vi "Create TCP Connection Handler.vi"(5 "TCPConnectionHandler in":refnum<class "TCPConnectionHandler.lvclass">, 8 "error in (no error)":errorcluster, 10 "NbConnections":refnum<user-event>, 11 "ServerRequest":refnum<queue>) -> (0 "error out":errorcluster, 3 "TCPConnectionHandler out":refnum<class "TCPConnectionHandler.lvclass">)   [LabVIEW 2013, in "MQTT_TCP.lvlib" / "TCPConnectionHandler.lvclass"]
uses:
  TCPConnectionHandler.lvclass
  MQTT_Base/Base Class/Request -- cluster.ctl
  <vilib>/LabVIEW Open Source Project/MQTT Control Packets/Control Packets/ControlPacket/ControlPacket.lvclass
  MQTT_Base/Base Class/Response -- cluster.ctl
  TCPConnectionHandler.lvclass/TCPConnectionHandler.ctl
  MQTT_Base/Base Class/MQTT_Base.lvclass
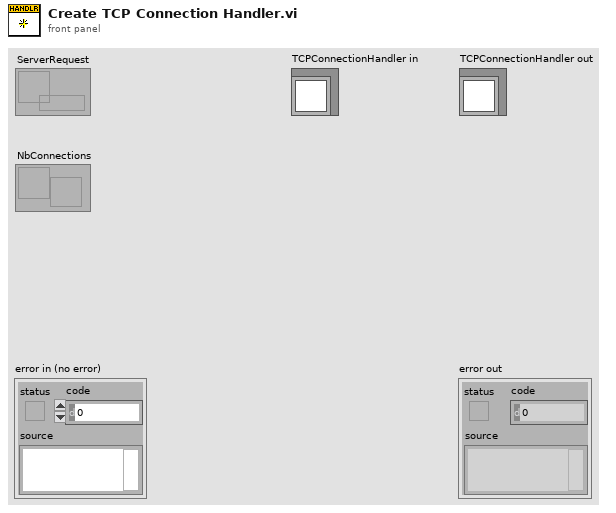
[diagram p1: front panel]
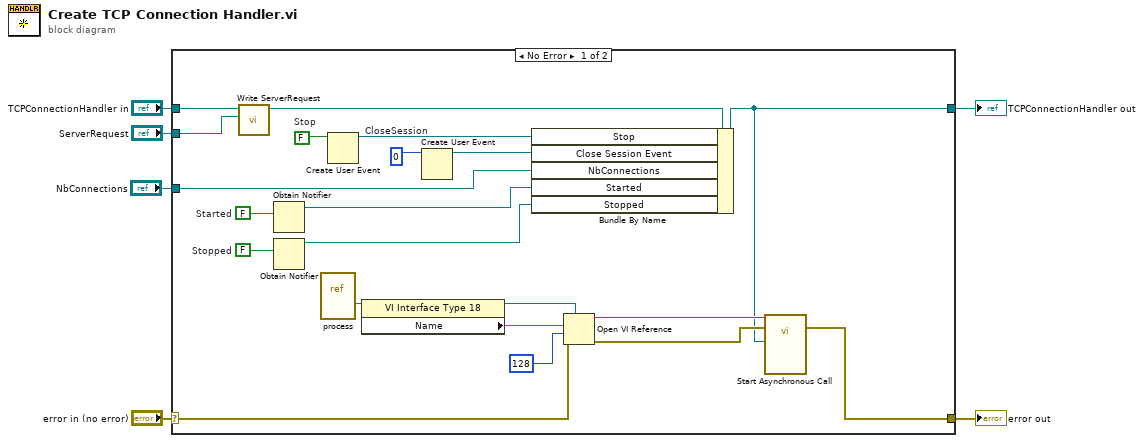
[diagram p0: block diagram]
diagram:
  n1 = case shown="No Error" "error in (no error)" {
    selector: "error in (no error)" -> [w8 w29]
    tunnel: [w7 w29] -> w5
    tunnel: [w16 w28] -> w3
    tunnel: "TCPConnectionHandler in" -> [w26 w28]
    tunnel: "ServerRequest" -> [w27 _]
    tunnel: "NbConnections" -> [w9 _]
    frame No Error {
      w12 = FALSE  # Stopped
      w13 = FALSE  # Started
      w15 = 0  # CloseSession
      w25 = FALSE  # Stop
      n2 = call "Write ServerRequest.vi"("ServerRequest"=w27, "TCPConnectionHandler in"=w26) -> ("TCPConnectionHandler out"=w23:refnum<class "TCPConnectionHandler.lvclass">)  [unwired: 9 in]
      n3 = Obtain Notifier(notification data type=w13) -> (notifier out=w11:refnum<notifier>)  [unwired: 3 in, 2 out]
      n4 = Obtain Notifier(notification data type=w12) -> (notifier out=w10:refnum<notifier>)  [unwired: 3 in, 2 out]
      n5 = vi-ref "process.vi"() -> (w22:refnum<vi>)
      n6 = Create User Event(user event datatype=w25) -> (user event=w24:refnum<user-event>)  [unwired: 1 in, 1 out]
      n7 = property class="VI Interface Type 18"(reference=w22) -> (reference out=w20:refnum<vi>, "Name"=w21:string)  [unwired: 1 in, 1 out]
      n8 = Create User Event(user event datatype=w15) -> (user event=w14:refnum<user-event>)  [unwired: 1 in, 1 out]
      n9 = Bundle By Name(cluster=w23, "Stop"=w24, "Close Session Event"=w14, "NbConnections"=w9, "Started"=w11, "Stopped"=w10) -> (w16:refnum<class "TCPConnectionHandler.lvclass">)
      n10 = Open VI Reference(type specifier VI Refnum (for type only)=w20, vi path=w21, options=128, error in (no error)=w8) -> (vi reference=w19:refnum<vi>, error out=w18:errorcluster)  [unwired: 2 in]
      n11 = call-by-ref "Start Asynchronous Call"(reference=w19, error in=w18, "TCPConnectionHandler in"=w16) -> (error out=w7:errorcluster)  [unwired: 9 in, 3 out]
    }
    frame Error {
    }
  }
  "error out" <- w5
  "TCPConnectionHandler out" <- w3
